vi "Get Notifier from Key.vi"(10 "Notifier Key":string) -> (1 "Payload":string, 2 "Frame":T1 {"CRC" format="%08x"; "Frame Header"."Options" format="%016b"; "Frame Header"."Time" format="%^<%I:%M:%S%3u %p\n%m/%d/%Y %Z>T"; "Frame Header"."Sync" format="%08x"}, 3 "Notifier":refnum<notifier>)   [LabVIEW 2021]
uses:
  Type Definitions/Data Frame.ctl
  Type Definitions/Data Frame Header.ctl
  Type Definitions/Payload Class.ctl
  Type Definitions/Device.ctl
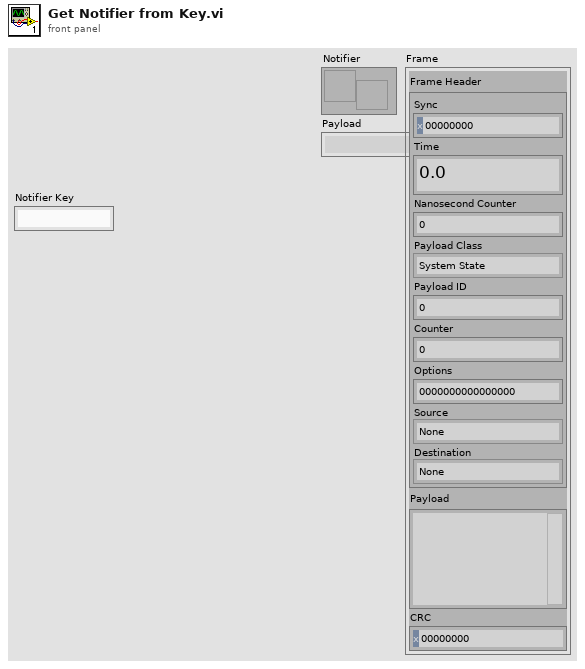
[diagram p1: front panel]
types:
  T1 = typedef "Data Frame.ctl" = cluster{"Frame Header":T2, "Payload":string, "CRC":u32}
  T2 = typedef "Data Frame Header.ctl" = cluster{"Sync":u32, "Time":dbl, "Nanosecond Counter":i64, "Payload Class":T3, "Payload ID":u16, "Counter":i32, "Options":u32, "Source":T4, "Destination":T4}
  T3 = typedef "Payload Class.ctl" = enum16{"System State", "Parameters", "Metadata", "Software Monitor", "Data", "Commands"}
  T4 = typedef "Device.ctl" = enum32{"None", "Exec", "Aux1", "Aux2", "Aux3"}
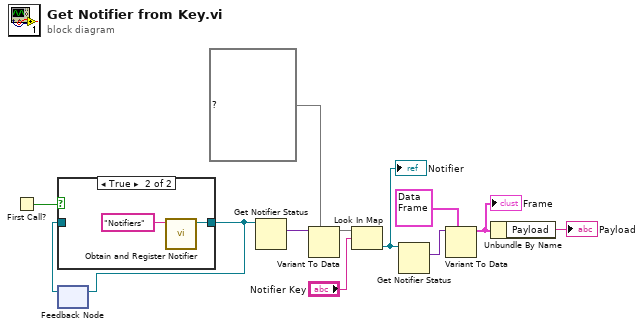
[diagram p0: block diagram]
diagram:
  n1 = First Call?() -> (First Call?: T/F=w3:bool)
  n2 = feedback #1() -> (w2:refnum<notifier>)  [unwired: 1 in]
  n3 = case shown="True" w3 {
    tunnel: [w13 w14] -> w1
    tunnel: w2 -> [w13 _]
    frame False {
    }
    frame True {
      n4 = call "Obtain and Register Notifier.vi"("name (unnamed)"="Notifiers") -> ("notifier out"=w14:refnum<notifier>)  [unwired: 8 in, 2 out]
    }
  }
  n5 = feedback-in #1(w1) -> ()
  n6 = Get Notifier Status(notifier=w1) -> (current notification=w9:variant)  [unwired: 1 in, 4 out]
  n7 = Variant To Data(type=map{string, refnum<notifier>} {} ("map"), Variant=w9) -> (data=w11:map{string, refnum<notifier>})  [unwired: 1 in, 1 out]
  n8 = Look In Map(map=w11, key="Notifier Key") -> (value=w8:refnum<notifier>)  [unwired: 1 in, 1 out]
  "Notifier" <- w8
  n9 = Get Notifier Status(notifier=w8) -> (current notification=w7:variant)  [unwired: 1 in, 4 out]
  n10 = Variant To Data(type=T1 {"Frame Header"={"Sync"=0, "Time"=0.0, "Nanosecond Counter"=0, "Payload Class"=enum."System State", "Payload ID"=0, "Counter"=0, "Options"=0, "Source"=enum."None", "Destination"=enum."None"}, "Payload"="", "CRC"=0} ("Frame"), Variant=w7) -> (data=w5:T1)  [unwired: 1 in, 1 out]
  "Frame" <- w5
  n11 = Unbundle By Name(w5) -> ("Payload"=→"Payload":string)
